vi "JudgeDataTrFreqAvialable.vi"(8 "错误输入（无错误）":errorcluster, 11 "需要设置的数据传输率":sgl) -> (0 "错误输出":errorcluster, 3 "返回值":i32)   [LabVIEW 2014]
uses:
  X86Dll/ZXUTConfigMgr.dll
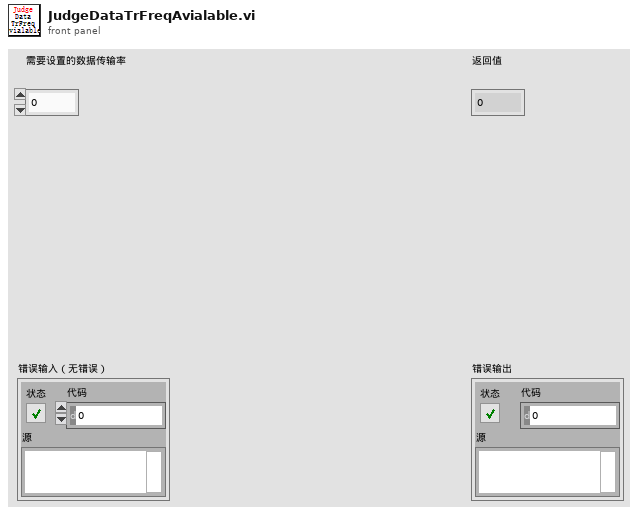
[diagram p1: front panel]
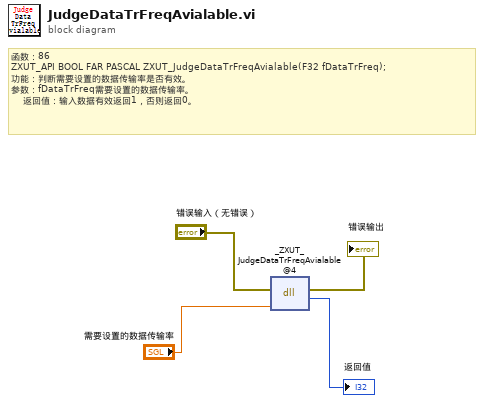
[diagram p0: block diagram]
diagram:
  # "函数：86\nZXUT_API BOOL\tFAR PASCAL ZXUT_JudgeDataTrFreqAvialable(F32 fDataTrFreq);\n功能：判断需要设置的数据传输率是否有效。\n参数：fDataTrFreq需要设置的数据传输率。\n\t   返回值：输入数据有效返回1，否则返回0。"
  n1 = dll-call lib="D:/Software/Utrasonic on-line monitoring/X86Dll/ZXUTConfigMgr.dll" fn="_ZXUT_JudgeDataTrFreqAvialable@4"(error in="错误输入（无错误）", "fDataTrFreq"="需要设置的数据传输率") -> (error out=→"错误输出":errorcluster, "返回值"=→"返回值":i32)  [unwired: 3 in, 1 out]
